vi "sub_GSlam_calc-observation-sigma.vi"() -> (3 "sigma":T1)   [LabVIEW 2019]
uses:
  <vilib>/Analysis/Matrix/Datatypes/RealMatrix.ctl
  Ctrl/cmd_common.ctl
  <vilib>/Analysis/Matrix/NI_Matrix.lvlib
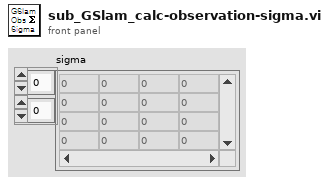
[diagram p1: front panel]
types:
  T1 = typedef "NI_Matrix.lvlib/RealMatrix.ctl" = dbl[][]
  T2 = typedef "cmd_common.ctl" = enum16{"read", "write"}
  T3 = cluster{"Q Sim":T1, "R Sim":T1, "DT":dbl, "SIM_TIME":dbl, "MAX_RANGE":dbl, "STATE_SIZE":i32, "C_SIGMA 1":dbl, "C_SIGMA 2":dbl, "C_SIGMA 3":dbl, "MAX_ITR":u32}
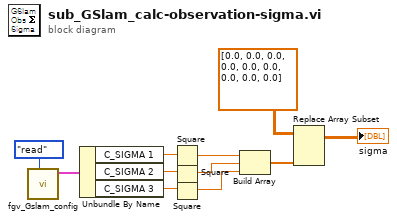
[diagram p0: block diagram]
diagram:
  n1 = call "fgv_Gslam_config.vi"("cmd"=cmd_common."read") -> ("G cofnig out"=w10:T3)  [unwired: 10 in]
  n2 = Unbundle By Name(w10) -> ("C_SIGMA 1"=w9:dbl, "C_SIGMA 2"=w8:dbl, "C_SIGMA 3"=w7:dbl)
  n3 = Square(x=w9) -> (x^2=w4:dbl)
  n4 = Square(x=w8) -> (x^2=w3:dbl)
  n5 = Square(x=w7) -> (x^2=w2:dbl)
  n6 = Build Array(w4, w3, w2) -> (w1:dbl[])
  n7 = Replace Array Subset(array=T1 [[0.0, 0.0, 0.0], [0.0, 0.0, 0.0], [0.0, 0.0, 0.0]] ("행렬"), new element=w1) -> (→"sigma":T1)  [unwired: 2 in]
